vi "Create Symbol Map Daemon Queue.vi"(8 "error in (no error)":errorcluster, 11 "TwinCAT ADS in":refnum<class "TwinCAT ADS.lvclass">) -> (0 "error out":errorcluster, 3 "TwinCAT ADS out":refnum<class "TwinCAT ADS.lvclass">)   [LabVIEW 2018, in "TwinCAT ADS.lvclass"]
uses:
  TwinCAT ADS.lvclass
  Controls/Daemon Message.ctl
  TwinCAT ADS.lvclass/TwinCAT ADS.ctl
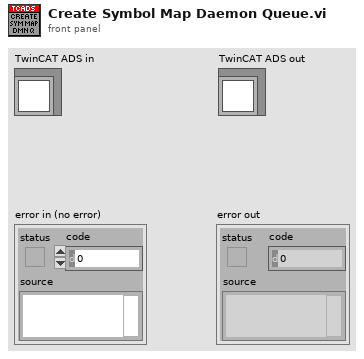
[diagram p1: front panel]
types:
  T1 = typedef "TwinCAT ADS.lvclass/Daemon Message.ctl" = cluster{"Symbol Name":string, "Occurrence":refnum<k4>}
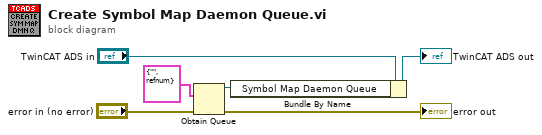
[diagram p0: block diagram]
diagram:
  n1 = Obtain Queue(element data type=T1 {"Symbol Name"="", "Occurrence"=refnum} ("Daemon Message"), error in (no error)="error in (no error)") -> (queue out=w2:refnum<queue>, error out=→"error out":errorcluster)  [unwired: 3 in, 1 out]
  n2 = Bundle By Name(cluster="TwinCAT ADS in", "Symbol Map Daemon Queue"=w2) -> (→"TwinCAT ADS out":refnum<class "TwinCAT ADS.lvclass">)
